vi "HRTF-Compute HRTFs.vi"(0 "State":T3, 2 "Progress":refnum<vi>, 5 "Window":T1, 9 "Desired Fs":dbl) -> (15 "error out":errorcluster)   [LabVIEW 2015]
uses:
  Typedefs/HRTF-State.ctl
  Typedefs/HRTF-Window.ctl
  Typedefs/HRTF-Window Type.ctl
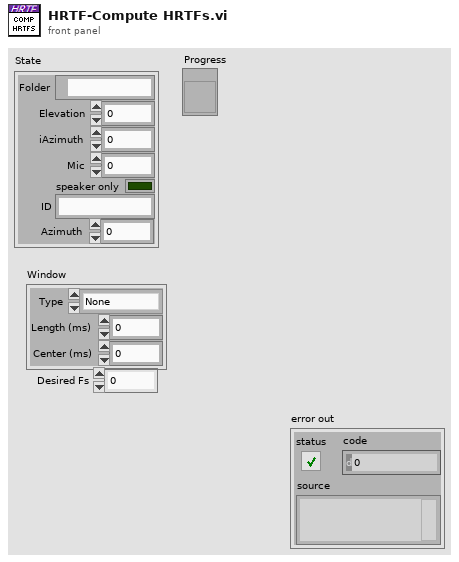
[diagram p1: front panel]
types:
  T1 = typedef "HRTF-Window.ctl" = cluster{"Type":T2, "Length (ms)":dbl, "Center (ms)":dbl}
  T2 = typedef "HRTF-Window Type.ctl" = enum16{"None", "Rectangle", "Hanning"}
  T3 = typedef "HRTF-State.ctl" = cluster{"Folder":path, "Elevation":dbl, "iAzimuth":i32, "Mic":i32, "speaker only":bool, "ID":string, "Azimuth":dbl}
  T4 = enum8{"Enabled", "Disabled", "Disabled and Grayed Out"}
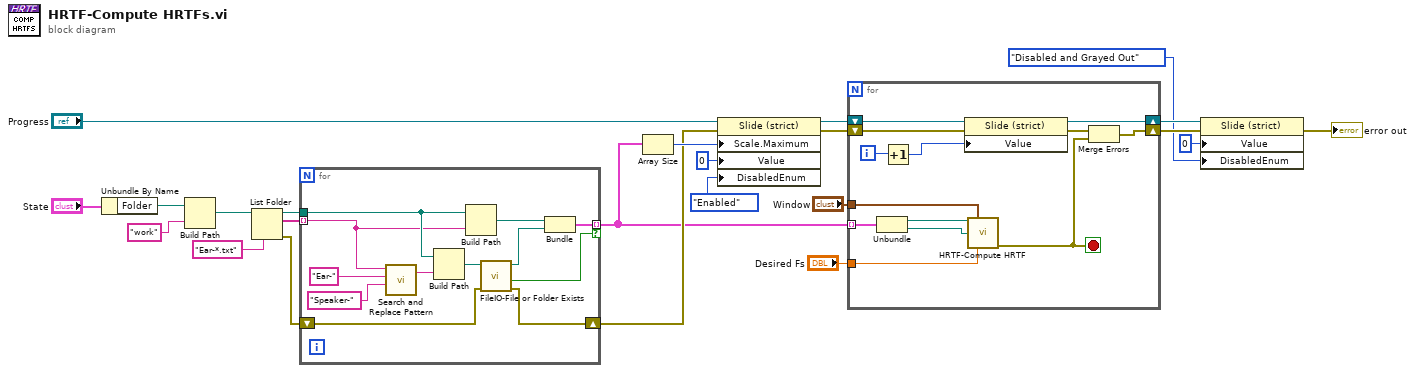
[diagram p0: block diagram]
diagram:
  n1 = Unbundle By Name("State") -> ("Folder"=w22:path)
  n2 = Build Path(base path=w22, name or relative path="work") -> (appended path=w20:path)
  n3 = List Folder(path=w20, pattern="Ear-*.txt") -> (path out=w18:path, filenames=w17:string[], error out=w16:errorcluster)  [unwired: 2 in, 1 out]
  n4 = for {
    tunnel: w18 -> [w31]
    tunnel: w17 -> [w30] mode=indexing
    tunnel: [w27] -> w11 mode=indexing if=w26
    shift-right: [w24] -> w12
    shift-left: w16 -> [w25]
    n5 = call <vilib>:"Search and Replace Pattern.vi"("string"=w30, "regular expression (\"\")"="Ear-" ("search string/char (-)"), "replace string (\"\")"="Speaker-" ("replace string (\"\")")) -> ("result string"=w33:string)  [unwired: 2 in, 1 out]
    n6 = Build Path(base path=w31, name or relative path=w33) -> (appended path=w32:path)
    n7 = Build Path(base path=w31, name or relative path=w30) -> (appended path=w29:path)
    n8 = call "FileIO-File or Folder Exists.vi"("error in (no error)"=w25, "path"=w32) -> ("error out"=w24:errorcluster, "Exists?"=w26:bool, "dup path"=w28:path)  [unwired: 6 in, 1 out]
    n9 = Bundle("appended path"=w29, "dup path"=w28) -> (w27:cluster{"appended path":path, "dup path":path})  [unwired: 1 in]
  }
  n10 = Array Size(array=w11) -> (size(s)=w14:i32)
  n11 = property class="Slide (strict)"(reference="Progress", error in=w12, "Scale.Maximum"=w14, "Value"=u8 0, "DisabledEnum"=T4."Enabled" ("Disabled")) -> (reference out=w10:refnum<vi>, error out=w9:errorcluster)
  n12 = for {
    tunnel: w11 -> [w43] mode=indexing
    shift-right: [w47] -> w7
    shift-left: w10 -> [w48]
    shift-right: [w36] -> w6
    shift-left: w9 -> [w46]
    tunnel: "Window" -> [w41]
    tunnel: "Desired Fs" -> [w39]
    i -> [w45]
    stop <- w37 stop-if-true
    n13 = Unbundle(w43) -> ("appended path"=w42:path, "dup path"=w40:path)
    n14 = Increment(x=w45) -> (x+1=w44:i32)
    n15 = property class="Slide (strict)"(reference=w48, error in=w46, "Value"=w44) -> (reference out=w47:refnum<vi>, error out=w38:errorcluster)
    n16 = call "HRTF-Compute HRTF.vi"("ear path"=w42, "Window"=w41, "speaker path"=w40, "Desired Fs"=w39) -> ("error out"=w37:errorcluster)  [unwired: 11 in]
    n17 = Merge Errors(w38, w37) -> (w36:errorcluster)
  }
  n18 = property class="Slide (strict)"(reference=w7, error in=w6, "Value"=u8 0, "DisabledEnum"=T4."Disabled and Grayed Out" ("Disabled")) -> (error out=→"error out":errorcluster)  [unwired: 1 out]
